vi "DTCDescriptor.FG.vi"(7 "Action":T1, 8 "error in (no error)":errorcluster, 10 "DTC":T2={"Descriptor"={"DTC Byte Length"=2, "Status Byte Length"=1, "Add Data Byte Length"=1, "Byte Order"=enum."Motorola"}, "Value.Code"=[], "Value.String"=[], "Value.J2012String"=[], "Status.Code"=[], "Status.String"=[]}, 11 "Device Item Ref in":T4 format="%.0x") -> (0 "error out":errorcluster, 2 "DTC descriptor":T2={"Descriptor"={"DTC Byte Length"=2, "Status Byte Length"=1, "Add Data Byte Length"=1, "Byte Order"=enum."Motorola"}, "Value.Code"=[], "Value.String"=[], "Value.J2012String"=[], "Status.Code"=[], "Status.String"=[]}, 3 "Device Item Ref out":T4=18446744073709551615 format="%.0x")   [LabVIEW 2019, in "Diagnostics Addon System Explorer.lvlib"]
uses:
  Diagnostics Addon System Explorer.lvlib
  <vilib>/NI VeriStand/Custom Device API/Custom Device Item Ref.ctl
  Shared/Types/DTC.Settings.ctl
  Shared/Types/DTC.Descriptor.ctl
  Types/FG.Action.ctl
  Shared/SubVIs/Constants.vi
  <vilib>/NI/NI VeriStand Advanced SysDef API/_SubVIs/SysDef.Property.Set.I32.vi
  <vilib>/NI/NI VeriStand Advanced SysDef API/_SubVIs/SysDef.Property.Set.U32.vi
  <vilib>/NI/NI VeriStand Advanced SysDef API/_SubVIs/SysDef.Property.Set.DBL.Array.vi
  <vilib>/NI/NI VeriStand Advanced SysDef API/_SubVIs/SysDef.Property.Set.String.Array.vi
  <vilib>/NI VeriStand/Custom Device API/Get Item Property (I32).vi
  <vilib>/NI VeriStand/Custom Device API/Get Item Property (U32).vi
  <vilib>/NI VeriStand/Custom Device API/Get Item Property (Double Array).vi
  <vilib>/NI VeriStand/Custom Device API/Get Item Property (String Array).vi
  Shared/Diagnostics Addon Shared.lvlib
  <vilib>/NI VeriStand/Custom Device API/Custom Device API.lvlib
  <vilib>/NI/NI VeriStand Advanced SysDef API/SysDef API/Advanced System Definition.lvlib
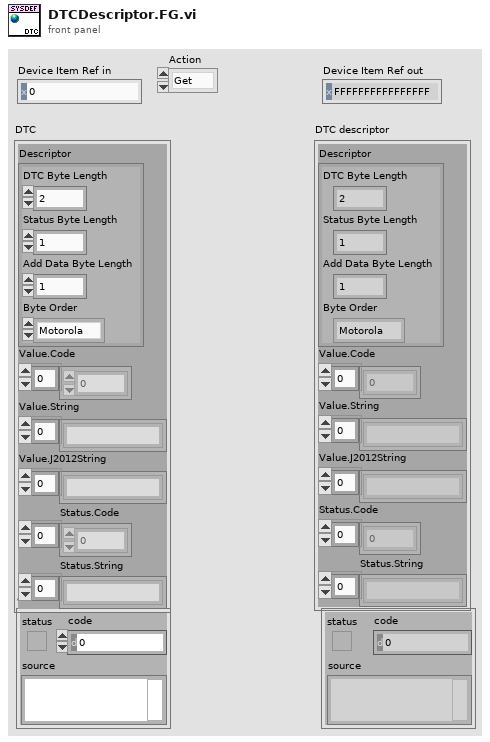
[diagram p1: front panel]
types:
  T1 = typedef "Diagnostics Addon System Explorer.lvlib/FG.Action.ctl" = enum16{"Get", "Set"}
  T2 = typedef "Diagnostics Addon Shared.lvlib/DTC.Settings.ctl" = cluster{"Descriptor":T3, "Value.Code":dbl[], "Value.String":string[], "Value.J2012String":string[], "Status.Code":dbl[], "Status.String":string[]}
  T3 = typedef "Diagnostics Addon Shared.lvlib/DTC.Descriptor.ctl" = cluster{"DTC Byte Length":i32, "Status Byte Length":i32, "Add Data Byte Length":i32, "Byte Order":enum16{"Motorola", "Intel"}}
  T4 = typedef "Custom Device API.lvlib/Custom Device Item Ref.ctl" = u64
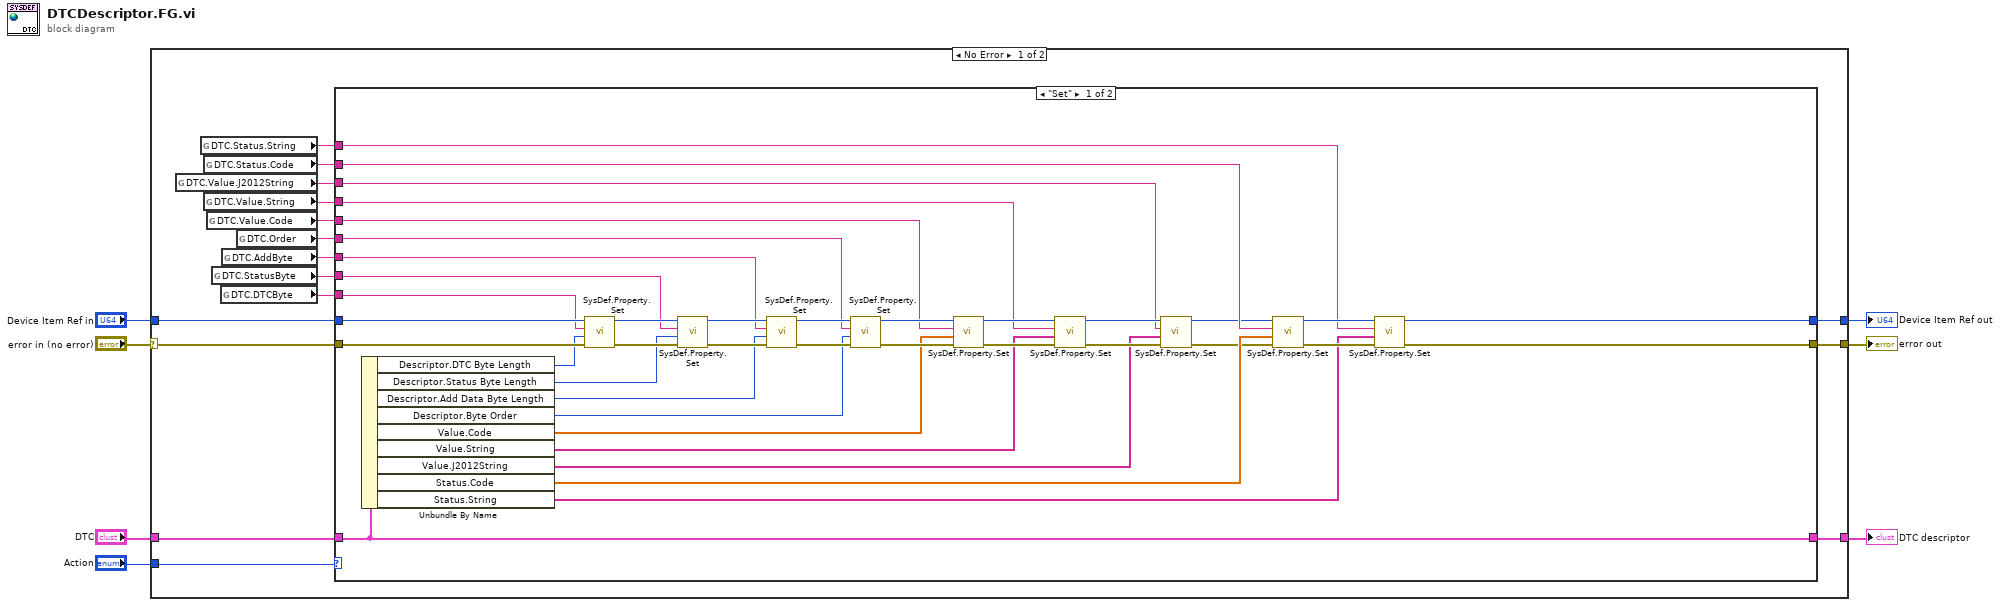
[diagram p0: block diagram]
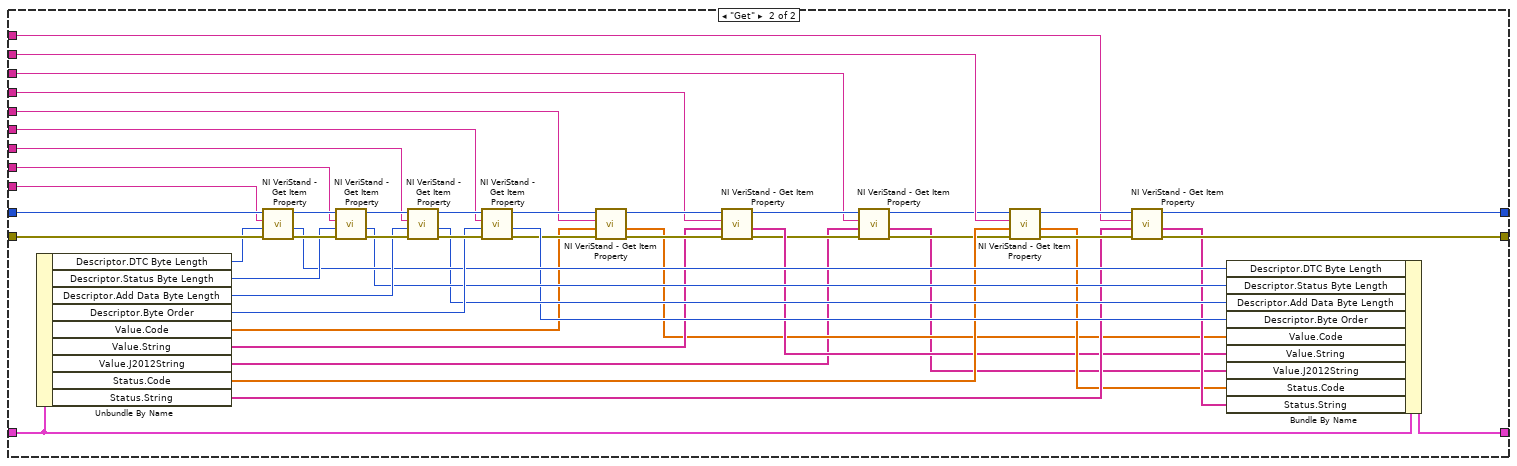
[diagram p2: hidden frame]
diagram:
  n1 = case shown="No Error" "error in (no error)" {
    selector: "error in (no error)" -> [w23 w112]
    tunnel: "Device Item Ref in" -> [w22 w113]
    tunnel: [w21 w113] -> w4
    tunnel: [w20 w112] -> w5
    tunnel: [w19 _] -> w3
    tunnel: "DTC" -> [w18 _]
    tunnel: "Action" -> [w17 _]
    frame No Error {
      n2 = global read "Constants.vi" "DTC.Value.J2012String"() -> (w8:string)
      n3 = global read "Constants.vi" "DTC.Status.String"() -> (w9:string)
      n4 = global read "Constants.vi" "DTC.Status.Code"() -> (w10:string)
      n5 = global read "Constants.vi" "DTC.Value.String"() -> (w11:string)
      n6 = global read "Constants.vi" "DTC.Value.Code"() -> (w12:string)
      n7 = global read "Constants.vi" "DTC.StatusByte"() -> (w15:string)
      n8 = global read "Constants.vi" "DTC.DTCByte"() -> (w16:string)
      n9 = global read "Constants.vi" "DTC.AddByte"() -> (w14:string)
      n10 = global read "Constants.vi" "DTC.Order"() -> (w13:string)
      n11 = case shown="\"Set\"" w17 {
        tunnel: w23 -> [w62 w111]
        tunnel: w22 -> [w61 w110]
        tunnel: [w38 w83] -> w21
        tunnel: [w40 w82] -> w20
        tunnel: [w60 w90] -> w19
        tunnel: w18 -> [w60 w95]
        tunnel: w16 -> [w48 w99]
        tunnel: w15 -> [w47 w98]
        tunnel: w14 -> [w46 w97]
        tunnel: w13 -> [w53 w96]
        tunnel: w12 -> [w33 w73]
        tunnel: w11 -> [w32 w72]
        tunnel: w10 -> [w31 w71]
        tunnel: w9 -> [w30 w70]
        tunnel: w8 -> [w25 w65]
        frame "Set" {
          n12 = Unbundle By Name(w60) -> ("Descriptor.DTC Byte Length"=w49:i32, "Descriptor.Status Byte Length"=w50:i32, "Descriptor.Add Data Byte Length"=w51:i32, "Descriptor.Byte Order"=w52:enum16{"Motorola", "Intel"}, "Value.Code"=w37:dbl[], "Value.String"=w36:string[], "Value.J2012String"=w24:string[], "Status.Code"=w35:dbl[], "Status.String"=w34:string[])
          n13 = call-poly <vilib>:"SysDef.Property.Set.vi"("error in (no error)"=w62, "Value"=w49, "Property Name"=w48, "nodeID"=w61) -> ("error out"=w59:errorcluster, "nodeID out"=w54:u64)  [unwired: 6 in]
          n14 = call-poly <vilib>:"SysDef.Property.Set.vi"("error in (no error)"=w59, "Value"=w50, "Property Name"=w47, "nodeID"=w54) -> ("error out"=w58:errorcluster, "nodeID out"=w55:u64)  [unwired: 6 in]
          n15 = call-poly <vilib>:"SysDef.Property.Set.vi"("error in (no error)"=w58, "Value"=w51, "Property Name"=w46, "nodeID"=w55) -> ("error out"=w57:errorcluster, "nodeID out"=w56:u64)  [unwired: 6 in]
          n16 = call-poly <vilib>:"SysDef.Property.Set.vi"("error in (no error)"=w57, "Value"=w52, "Property Name"=w53, "nodeID"=w56) -> ("error out"=w44:errorcluster, "nodeID out"=w45:u64)  [unwired: 6 in]
          n17 = call-poly <vilib>:"SysDef.Property.Set.vi"("error in (no error)"=w44, "Value"=w37, "Property Name"=w33, "nodeID"=w45) -> ("error out"=w43:errorcluster, "nodeID out"=w42:u64)  [unwired: 6 in]
          n18 = call-poly <vilib>:"SysDef.Property.Set.vi"("error in (no error)"=w43, "Value"=w36, "Property Name"=w32, "nodeID"=w42) -> ("error out"=w27:errorcluster, "nodeID out"=w29:u64)  [unwired: 6 in]
          n19 = call-poly <vilib>:"SysDef.Property.Set.vi"("error in (no error)"=w27, "Value"=w24, "Property Name"=w25, "nodeID"=w29) -> ("error out"=w26:errorcluster, "nodeID out"=w28:u64)  [unwired: 6 in]
          n20 = call-poly <vilib>:"SysDef.Property.Set.vi"("error in (no error)"=w26, "Value"=w35, "Property Name"=w31, "nodeID"=w28) -> ("error out"=w41:errorcluster, "nodeID out"=w39:u64)  [unwired: 6 in]
          n21 = call-poly <vilib>:"SysDef.Property.Set.vi"("error in (no error)"=w41, "Value"=w34, "Property Name"=w30, "nodeID"=w39) -> ("error out"=w40:errorcluster, "nodeID out"=w38:u64)  [unwired: 6 in]
        }
        frame "Get" {
          n22 = Unbundle By Name(w95) -> ("Descriptor.DTC Byte Length"=w103:i32, "Descriptor.Status Byte Length"=w102:i32, "Descriptor.Add Data Byte Length"=w101:i32, "Descriptor.Byte Order"=w100:enum16{"Motorola", "Intel"}, "Value.Code"=w81:dbl[], "Value.String"=w80:string[], "Value.J2012String"=w64:string[], "Status.Code"=w79:dbl[], "Status.String"=w78:string[])
          n23 = call-poly <vilib>:"NI VeriStand - Get Item Property.vi"("error in (no error)"=w111, "Default Value"=w103, "Property Name"=w99, "Item Ref in"=w110) -> ("error out"=w109:errorcluster, "Value"=w94:i32, "Item Ref out"=w106:T4)  [unwired: 4 in, 1 out]
          n24 = call-poly <vilib>:"NI VeriStand - Get Item Property.vi"("error in (no error)"=w109, "Default Value"=w102, "Property Name"=w98, "Item Ref in"=w106) -> ("error out"=w108:errorcluster, "Value"=w93:i32, "Item Ref out"=w105:T4)  [unwired: 4 in, 1 out]
          n25 = call-poly <vilib>:"NI VeriStand - Get Item Property.vi"("error in (no error)"=w108, "Default Value"=w101, "Property Name"=w97, "Item Ref in"=w105) -> ("error out"=w107:errorcluster, "Value"=w92:i32, "Item Ref out"=w104:T4)  [unwired: 4 in, 1 out]
          n26 = call-poly <vilib>:"NI VeriStand - Get Item Property.vi"("error in (no error)"=w107, "Default Value"=w100, "Property Name"=w96, "Item Ref in"=w104) -> ("error out"=w85:errorcluster, "Value"=w91:u32, "Item Ref out"=w84:T4)  [unwired: 4 in, 1 out]
          n27 = call-poly <vilib>:"NI VeriStand - Get Item Property.vi"("error in (no error)"=w85, "Default Value"=w81, "Property Name"=w73, "Item Ref in"=w84) -> ("error out"=w86:errorcluster, "Value"=w74:dbl[], "Item Ref out"=w88:T4)  [unwired: 4 in, 1 out]
          n28 = call-poly <vilib>:"NI VeriStand - Get Item Property.vi"("error in (no error)"=w86, "Default Value"=w80, "Property Name"=w72, "Item Ref in"=w88) -> ("error out"=w68:errorcluster, "Value"=w75:string[], "Item Ref out"=w69:T4)  [unwired: 4 in, 1 out]
          n29 = call-poly <vilib>:"NI VeriStand - Get Item Property.vi"("error in (no error)"=w68, "Default Value"=w64, "Property Name"=w65, "Item Ref in"=w69) -> ("error out"=w67:errorcluster, "Value"=w63:string[], "Item Ref out"=w66:T4)  [unwired: 4 in, 1 out]
          n30 = call-poly <vilib>:"NI VeriStand - Get Item Property.vi"("error in (no error)"=w67, "Default Value"=w79, "Property Name"=w71, "Item Ref in"=w66) -> ("error out"=w87:errorcluster, "Value"=w76:dbl[], "Item Ref out"=w89:T4)  [unwired: 4 in, 1 out]
          n31 = call-poly <vilib>:"NI VeriStand - Get Item Property.vi"("error in (no error)"=w87, "Default Value"=w78, "Property Name"=w70, "Item Ref in"=w89) -> ("error out"=w82:errorcluster, "Value"=w77:string[], "Item Ref out"=w83:T4)  [unwired: 4 in, 1 out]
          n32 = Bundle By Name(cluster=w95, "Descriptor.DTC Byte Length"=w94, "Descriptor.Status Byte Length"=w93, "Descriptor.Add Data Byte Length"=w92, "Descriptor.Byte Order"=w91, "Value.Code"=w74, "Value.String"=w75, "Value.J2012String"=w63, "Status.Code"=w76, "Status.String"=w77) -> (w90:T2)
        }
      }
    }
    frame Error {
    }
  }
  "error out" <- w5
  "Device Item Ref out" <- w4
  "DTC descriptor" <- w3
